vi "Init Events.vi"(8 "error in (no error)":errorcluster, 11 "BetterSearch in":refnum<class "BetterSearch.lvclass">) -> (0 "error out":errorcluster, 3 "BetterSearch out":refnum<class "BetterSearch.lvclass">)   [LabVIEW 2016, in "Better Search.lvlib" / "BetterSearch.lvclass"]
uses:
  BetterSearch.lvclass
  Data Types/Search Context.ctl
  Better Search.lvlib
  Search/Search.lvclass
  Search Result/Search Result.lvclass
  Search Result.ctl
  Data Types/Start Search Type.ctl
  Data Types/Type Reflection Item.ctl
  Search Progress.ctl
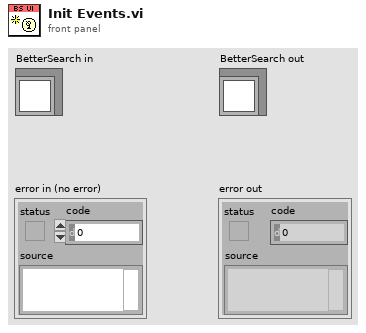
[diagram p1: front panel]
types:
  T1 = typedef "Better Search.lvlib/Search Progress.ctl" = cluster{"Complete":bool, "Label":string}
  T2 = typedef "Better Search.lvlib/Search Result.ctl" = cluster{"Search":refnum<class "Search.lvclass">, "Result":refnum<class "Search Result.lvclass">}
  T3 = typedef "Better Search.lvlib/Search Context.ctl" = cluster{"Type ID":string, "VI Refnum":refnum<vi>, "Starting Text":string, "Shift?":bool, "App Ref":refnum<vi>, "Start Search Type":T4, "Item Graph":T5[], "Variant":variant}
  T4 = typedef "Better Search.lvlib/Start Search Type.ctl" = enum16{"Auto", "Text", "Data Type", "Bundle"}
  T5 = typedef "Better Search.lvlib/Type Reflection Item.ctl" = cluster{"Parent":i32, "Depth":i32, "Children":i32[], "Skip":bool, "Name":string, "Type":variant, "TypeID":string}
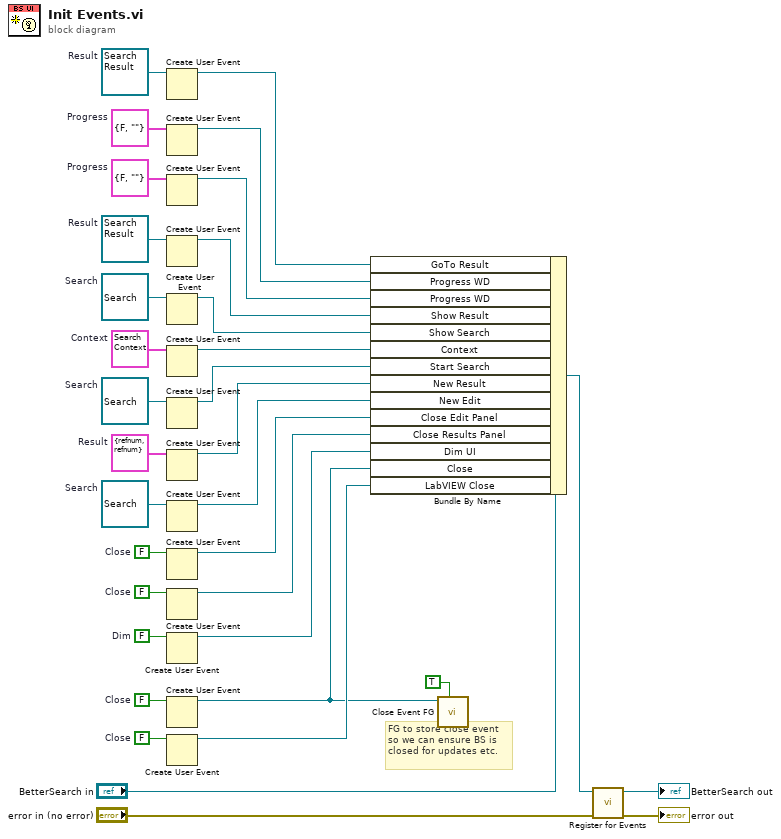
[diagram p0: block diagram]
diagram:
  w2 = refnum<class "Search Result.lvclass"> refnum  # Result
  w6 = T1 {"Complete"=FALSE, "Label"=""}  # Progress
  w8 = T1 {"Complete"=FALSE, "Label"=""}  # Progress
  w10 = FALSE  # Close
  w11 = FALSE  # Close
  w13 = FALSE  # Dim
  w15 = refnum<class "Search Result.lvclass"> refnum  # Result
  w17 = refnum<class "Search.lvclass"> refnum  # Search
  w24 = FALSE  # Close
  w25 = FALSE  # Close
  w30 = refnum<class "Search.lvclass"> refnum  # Search
  w31 = T2 {"Search"=refnum, "Result"=refnum}  # Result
  w32 = refnum<class "Search.lvclass"> refnum  # Search
  w33 = T3 {"Type ID"="", "VI Refnum"=refnum, "Starting Text"="", "Shift?"=FALSE, "App Ref"=refnum, "Start Search Type"=enum."Auto", "Item Graph"=[], "Variant"=variant}  # Context
  # "FG to store close event so we can ensure BS is closed for updates etc."
  n1 = Create User Event(user event datatype=w2) -> (user event=w1:refnum<user-event>)  [unwired: 1 in, 1 out]
  n2 = Create User Event(user event datatype=w6) -> (user event=w5:refnum<user-event>)  [unwired: 1 in, 1 out]
  n3 = Create User Event(user event datatype=w8) -> (user event=w7:refnum<user-event>)  [unwired: 1 in, 1 out]
  n4 = Create User Event(user event datatype=w15) -> (user event=w14:refnum<user-event>)  [unwired: 1 in, 1 out]
  n5 = Create User Event(user event datatype=w17) -> (user event=w16:refnum<user-event>)  [unwired: 1 in, 1 out]
  n6 = Create User Event(user event datatype=w33) -> (user event=w29:refnum<user-event>)  [unwired: 1 in, 1 out]
  n7 = Create User Event(user event datatype=w32) -> (user event=w28:refnum<user-event>)  [unwired: 1 in, 1 out]
  n8 = Create User Event(user event datatype=w31) -> (user event=w27:refnum<user-event>)  [unwired: 1 in, 1 out]
  n9 = Create User Event(user event datatype=w30) -> (user event=w26:refnum<user-event>)  [unwired: 1 in, 1 out]
  n10 = Create User Event(user event datatype=w25) -> (user event=w23:refnum<user-event>)  [unwired: 1 in, 1 out]
  n11 = Create User Event(user event datatype=w24) -> (user event=w22:refnum<user-event>)  [unwired: 1 in, 1 out]
  n12 = Create User Event(user event datatype=w13) -> (user event=w12:refnum<user-event>)  [unwired: 1 in, 1 out]
  n13 = Create User Event(user event datatype=w11) -> (user event=w4:refnum<user-event>)  [unwired: 1 in, 1 out]
  n14 = Create User Event(user event datatype=w10) -> (user event=w9:refnum<user-event>)  [unwired: 1 in, 1 out]
  n15 = Bundle By Name(cluster="BetterSearch in", "GoTo Result"=w1, "Progress WD"=w5, "Progress WD"=w7, "Show Result"=w14, "Show Search"=w16, "Context"=w29, "Start Search"=w28, "New Result"=w27, "New Edit"=w26, "Close Edit Panel"=w23, "Close Results Panel"=w22, "Dim UI"=w12, "Close"=w4, "LabVIEW Close"=w9) -> (w20:refnum<class "BetterSearch.lvclass">)
  n16 = call "Close Event FG.vi"("Set (F)"=TRUE, "Close In"=w4) -> ()  [unwired: 9 in, 1 out]
  n17 = call "Register for Events.vi"("error in (no error)"="error in (no error)", "BetterSearch in"=w20) -> ("error out"=→"error out":errorcluster, "BetterSearch out"=→"BetterSearch out":refnum<class "BetterSearch.lvclass">)  [unwired: 8 in]
